vi "default_config_OSC.vi"(0 "VISA resource in":refnum<visa-resource-name>="OSC", 11 "error in (no error)":errorcluster) -> (4 "VISA resource name out":refnum<visa-resource-name>, 15 "error out":errorcluster)   [LabVIEW 2012]
doc: "Sets OCS to its default settings for the chirped pulse measurement. The time base (time/div, sample rate, etc.) is not changed."
uses:
  controls/sampling_rate.ctl
  controls/scale.ctl
  global.vi
  libaries/Tektronix 7000 Series/Public/Configure/Configure Trigger (Edge).vi
  libaries/Tektronix 7000 Series/Tektronix 7000 Series.lvlib
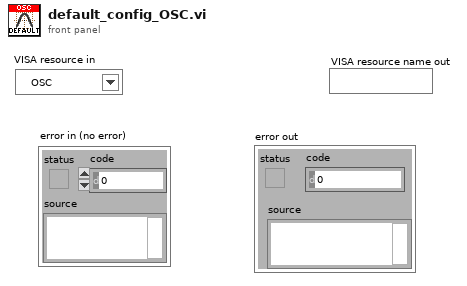
[diagram p1: front panel]
types:
  T1 = typedef "scale.ctl" = dbl
  T2 = typedef "sampling_rate.ctl" = ext
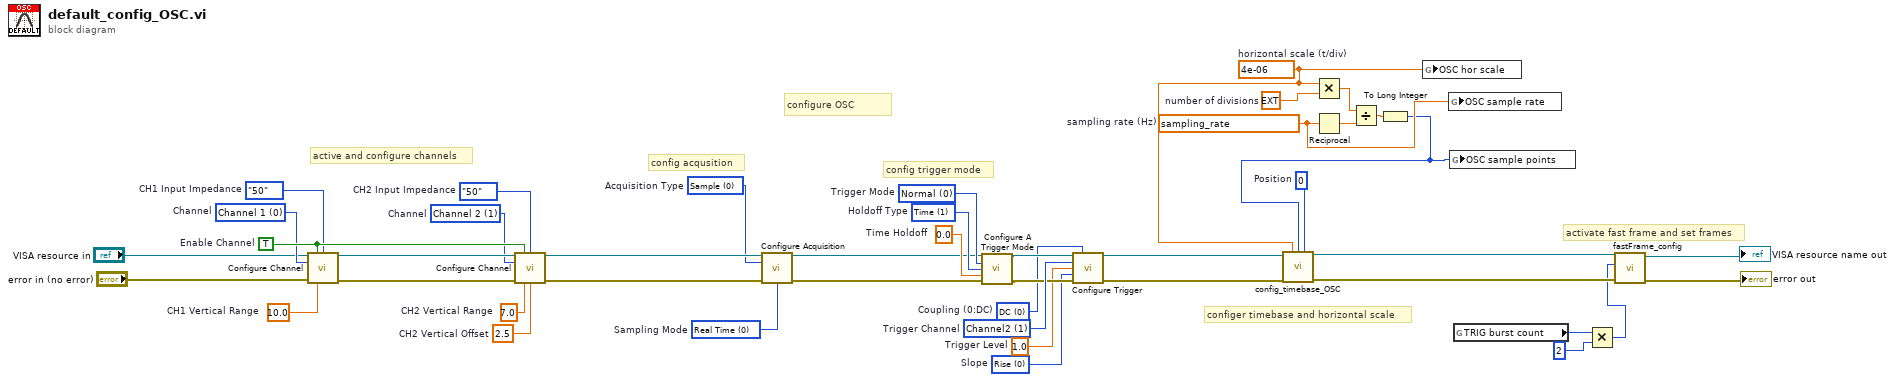
[diagram p0: block diagram]
diagram:
  w10 = u16 0 items=["Real Time", "Interpolater", "Equivalent"]  # Sampling Mode
  w11 = u16 0 items=["Sample", "Peak Detect", "Hi Res", "Average", "Envelope", "WfmDB"]  # Acquisition Type
  w18 = enum16{"1M", "50"}."50"  # CH1 Input Impedance
  w19 = enum16{"1M", "50"}."50"  # CH2 Input Impedance
  w20 = 10.0  # CH1 Vertical Range
  w21 = 2.5  # CH2 Vertical Offset
  w22 = 7.0  # CH2 Vertical Range
  w24 = u16 1 items=["Channel 1", "Channel 2", "Channel 3", "Channel 4", "Math 1", "Math 2", "Math 3", "Math 4", "Reference 1", "Reference 2", "Reference 3", "Reference 4"]  # Channel
  w25 = TRUE  # Enable Channel
  w23 = u16 0 items=["Channel 1", "Channel 2", "Channel 3", "Channel 4", "Math 1", "Math 2", "Math 3", "Math 4", "Reference 1", "Reference 2", "Reference 3", "Reference 4"]  # Channel
  w8 = T1 4e-06 items=["400ns/div"=4e-07, "1µs/div"=1e-06, "2µs/div"=2e-06, "4µs/div"=4e-06, "10µs/div"=1e-05, "20µs/div"=2e-05]  # horizontal scale (t/div)
  w28 = T2 5000000000.0 items=["20 GHz (50ps/sample)", "10 GHz (100ps/sample)", "5.0 GHz (200ps/sample)", "2.5 GHz (400ps/sample)", "1.25 GHz (0.8ns/sample)", "0.5 GHz (2ns/sample)"]  # sampling rate (Hz)
  w32 = ext 10.0  # number of divisions
  w36 = u16 0 items=["DC", "AC", "Hf Reject", "Lf Reject", "Noise Rej", "Atrigger"]  # Coupling (0:DC)
  w37 = u16 0 items=["Rise", "Fall", "Either"]  # Slope
  w38 = 1.0  # Trigger Level
  w35 = u16 0 items=["Normal", "Auto"]  # Trigger Mode
  w41 = 0.0  # Time Holdoff
  w42 = u16 1 items=["Auto", "Time", "Random"]  # Holdoff Type
  w43 = u16 1 items=["Channel1"=0, "Channel2"=1, "Channel3"=2, "Channel4"=3, "Aux"=12, "Line"=13, "Digital Channel0"=14, "Digital Channel1"=15, "Digital Channel2"=16, "Digital Channel3"=17, "Digital Channel4"=18, "Digital Chennel5"=19, "Digital Channel6"=20, "Digital Channel7"=21, "Digital Channel8"=22, "Digital Channel9"=23, "Digital Channel10"=24, "Digital Channel11"=25, "Digital Channel12"=26, "Digital Channel13"=27, "Digital Channel14"=28, "Digital Channel15"=29]  # Trigger Channel
  w44 = 0  # Position
  # "activate fast frame and set frames"
  # "config acqusition"
  # "active and configure channels"
  # "configer timebase and horizontal scale"
  # "config trigger mode"
  # "configure OSC"
  n1 = call "Configure Channel.vi"("VISA resource name"="VISA resource in", "Enable Channel (T: Enable)"=w25, "Input Impedance (0: 1M ohm)"=w18, "Channel (0: Channel 1)"=w23, "error in (no error)"="error in (no error)", "Vertical Range (10.0 V)"=w20) -> ("VISA resource name out"=w26:refnum<visa-resource-name>, "error out"=w27:errorcluster)  [unwired: 8 in]
  n2 = call "Configure Channel.vi"("VISA resource name"=w26, "Enable Channel (T: Enable)"=w25, "Input Impedance (0: 1M ohm)"=w19, "Channel (0: Channel 1)"=w24, "error in (no error)"=w27, "Vertical Range (10.0 V)"=w22, "Vertical Offset (0.0 V)"=w21) -> ("VISA resource name out"=w15:refnum<visa-resource-name>, "error out"=w14:errorcluster)  [unwired: 7 in]
  n3 = call "Configure Acquisition.vi"("VISA resource name"=w15, "Acquisition Type (0:Sample)"=w11, "error in (no error)"=w14, "Sampling Modes (Real Time)"=w10) -> ("VISA resource name out"=w13:refnum<visa-resource-name>, "error out"=w12:errorcluster)  [unwired: 10 in]
  n4 = call "Configure A Trigger Mode.vi"("VISA resource name"=w13, "Trigger Mode (0:Normal)"=w35, "Holdoff Type (0:Auto)"=w42, "Time Holdoff (1us)"=w41, "error in (no error)"=w12) -> ("VISA resource name out"=w40:refnum<visa-resource-name>, "error out"=w39:errorcluster)  [unwired: 9 in]
  n5 = call-poly "Configure Trigger.vi"("VISA resource name"=w40, "Coupling (0:DC)"=w36, "Source (0:Channel1)"=w43, "Trigger Level (0.0V)"=w38, "Slope (0:Rise)"=w37, "error in (no error)"=w39) -> ("VISA resource name out"=w34:refnum<visa-resource-name>, "error out"=w33:errorcluster)  [unwired: 8 in]
  n6 = Multiply(x=w8, y=w32) -> (x*y=w29:ext)
  n7 = Reciprocal(x=w28) -> (1/x=w31:T2)
  n8 = Divide(x=w29, y=w31) -> (x/y=w30:T2)
  n9 = To Long Integer(number=w30) -> (32bit integer=w9:i32)
  n10 = call "config_timebase_OSC.vi"("VISA resource name"=w34, "hor scale"=w8, "resolution"=w9, "Position"=w44, "error in (no error)"=w33) -> ("VISA resource name out"=w7:refnum<visa-resource-name>, "error out"=w6:errorcluster)  [unwired: 9 in]
  n11 = global write "global.vi" "OSC hor scale"(w8) -> ()
  n12 = global write "global.vi" "OSC sample rate"(w28) -> ()
  n13 = global write "global.vi" "OSC sample points"(w9) -> ()
  n14 = global read "global.vi" "TRIG burst count"() -> (w2:i32)
  n15 = Multiply(x=w2, y=2) -> (x*y=w1:i32)
  n16 = call "fastFrame_config.vi"("error in (no error)"=w6, "fast frame count"=w1, "VISA resource name"=w7) -> ("error out"=→"error out":errorcluster, "VISA resource name out"=→"VISA resource name out":refnum<visa-resource-name>)  [unwired: 7 in]
